vi "Create Exit Event.vi"() -> (1 "User Event Out":refnum<user-event>, 3 "Event Registration Refnum":refnum<event-registration>)   [LabVIEW 2012]
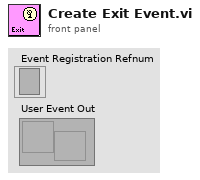
[diagram p1: front panel]
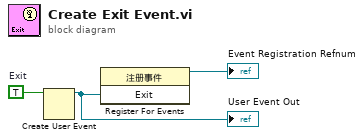
[diagram p0: block diagram]
diagram:
  w1 = TRUE  # Exit
  n1 = Create User Event(user event datatype=w1) -> (user event=w2:refnum<user-event>)  [unwired: 1 in, 1 out]
  "User Event Out" <- w2
  n2 = register-events(w2) -> (reference out=→"Event Registration Refnum":refnum<event-registration>)  [unwired: 2 in, 1 out]
